vi "GetTargetPose.vi"() -> ()   [LabVIEW 2018]
uses:
  Math/Vector/Vector3D.ctl
  Math/Pose/Pose3D.ctl
  Math/Vector/Vector3DtoVector2D_XY.vi
panel:
  out "TopMiddleTarget":T1
  out "Right Target Distance":dbl
  out "Left Target Distance":dbl
  out "Angle":dbl
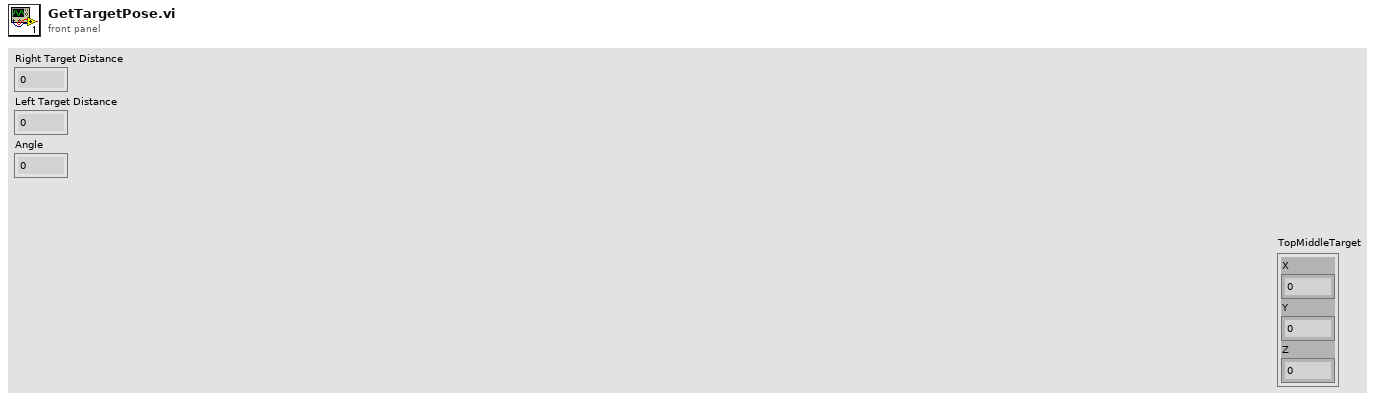
[diagram p1: front panel]
types:
  T1 = typedef "Vector3D.ctl" = cluster{"X":dbl, "Y":dbl, "Z":dbl}
  T2 = typedef "Pose3D.ctl" = cluster{"X":dbl, "Y":dbl, "Z":dbl, "Rotation":dbl}
  T3 = typedef "Vector2D.ctl" = cluster{"X":dbl, "Y":dbl}
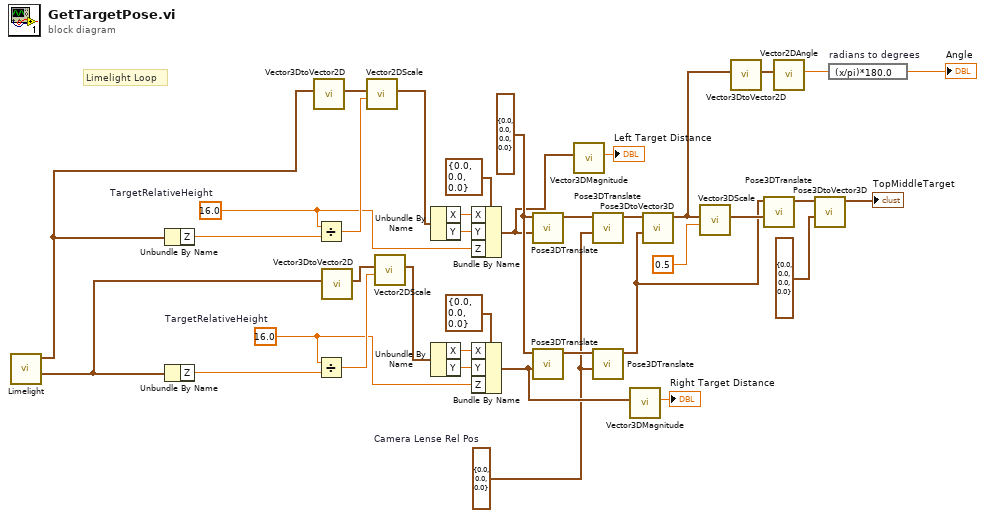
[diagram p0: block diagram]
diagram:
  w1 = 16.0  # TargetRelativeHeight
  w2 = 16.0  # TargetRelativeHeight
  w3 = T1 {"X"=0.0, "Y"=0.0, "Z"=0.0}  # Camera Lense Rel Pos
  w29 = T2 {"X"=0.0, "Y"=0.0, "Z"=0.0, "Rotation"=0.0} ("Starting Pose")
  # "Limelight Loop"
  n1 = call "Limelight.vi"() -> ("RightTargetNorm"=w12:T1, "LeftTargetNorm"=w17:T1)  [unwired: 10 in]
  n2 = Unbundle By Name(w17) -> ("Z"=w36:dbl)
  n3 = Unbundle By Name(w12) -> ("Z"=w35:dbl)
  n4 = call-poly "Vector3DtoVector2D.vi"("Vector3D"=w17) -> ("Vector2D"=w16:T3)  [unwired: 10 in]
  n5 = Divide(x=w1, y=w36) -> (x/y=w15:dbl)
  n6 = Divide(x=w2, y=w35) -> (x/y=w8:dbl)
  n7 = call-poly "Vector3DtoVector2D.vi"("Vector3D"=w12) -> ("Vector2D"=w13:T3)  [unwired: 10 in]
  n8 = call "Vector2DScale.vi"("Scale Factor"=w15, "Vector"=w16) -> ("Scaled Vector"=w14:T3)  [unwired: 9 in]
  n9 = call "Vector2DScale.vi"("Scale Factor"=w8, "Vector"=w13) -> ("Scaled Vector"=w11:T3)  [unwired: 9 in]
  n10 = Unbundle By Name(w14) -> ("X"=w33:dbl, "Y"=w32:dbl)
  n11 = Unbundle By Name(w11) -> ("X"=w10:dbl, "Y"=w9:dbl)
  n12 = Bundle By Name(cluster=T1 {"X"=0.0, "Y"=0.0, "Z"=0.0} ("Vector3D"), "X"=w33, "Y"=w32, "Z"=w1) -> (w21:T1)
  n13 = Bundle By Name(cluster=T1 {"X"=0.0, "Y"=0.0, "Z"=0.0} ("Vector3D"), "X"=w10, "Y"=w9, "Z"=w2) -> (w20:T1)
  n14 = call "Pose3DTranslate.vi"("Translation Vector"=w21, "Starting Pose"=w29) -> ("Resulting Pose"=w31:T2)  [unwired: 9 in]
  n15 = call "Pose3DTranslate.vi"("Translation Vector"=w20, "Starting Pose"=w29) -> ("Resulting Pose"=w30:T2)  [unwired: 9 in]
  n16 = call "Vector3DMagnitude.vi"("Vector3D"=w21) -> ("Magnitude"=→"Left Target Distance":dbl)  [unwired: 10 in]
  n17 = call "Pose3DTranslate.vi"("Translation Vector"=w3, "Starting Pose"=w31) -> ("Resulting Pose"=w26:T2)  [unwired: 9 in]
  n18 = call "Pose3DTranslate.vi"("Translation Vector"=w3, "Starting Pose"=w30) -> ("Resulting Pose"=w25:T2)  [unwired: 9 in]
  n19 = call "Vector3DMagnitude.vi"("Vector3D"=w20) -> ("Magnitude"=→"Right Target Distance":dbl)  [unwired: 10 in]
  n20 = call "Pose3DtoVector3D.vi"("Tail"=w25, "Nose"=w26) -> ("Vector3D"=w7:T1)  [unwired: 9 in]
  n21 = call "Vector3DScale.vi"("Scale Factor"=0.5, "Vector3D"=w7) -> ("Scaled Vector"=w27:T1)  [unwired: 9 in]
  n22 = call-poly "Vector3DtoVector2D.vi"("Vector3D"=w7) -> ("Vector2D"=w6:T3)  [unwired: 10 in]
  n23 = call "Pose3DTranslate.vi"("Translation Vector"=w27, "Starting Pose"=w25) -> ("Resulting Pose"=w24:T2)  [unwired: 9 in]
  n24 = call "Vector2DAngle.vi"("Vector2D"=w6) -> ("Angle"=w5:dbl)  [unwired: 10 in]
  n25 = call "Pose3DtoVector3D.vi"("Tail"=T2 {"X"=0.0, "Y"=0.0, "Z"=0.0, "Rotation"=0.0} ("Starting Pose"), "Nose"=w24) -> ("Vector3D"=→"TopMiddleTarget":T1)  [unwired: 9 in]
  n26 = expression code="(x/pi)*180.0" "radians to degrees"(w5) -> (→"Angle":dbl)
